vi "Get Channel Groups.vi"(8 "error in":errorcluster, 10 "Channel JSON List":string[](array[string]), 11 "Channel Type List":string[](array[string])) -> (0 "error out":errorcluster, 3 "ChannelGroups":T1)   [LabVIEW 2026, in "Template Deployment Hooks.lvlib"]
uses:
  Template Deployment Hooks.lvlib
  <vilib>/JDP Science/JSONtext/JSONtext.lvlib
  Types/Channel Mode.ctl
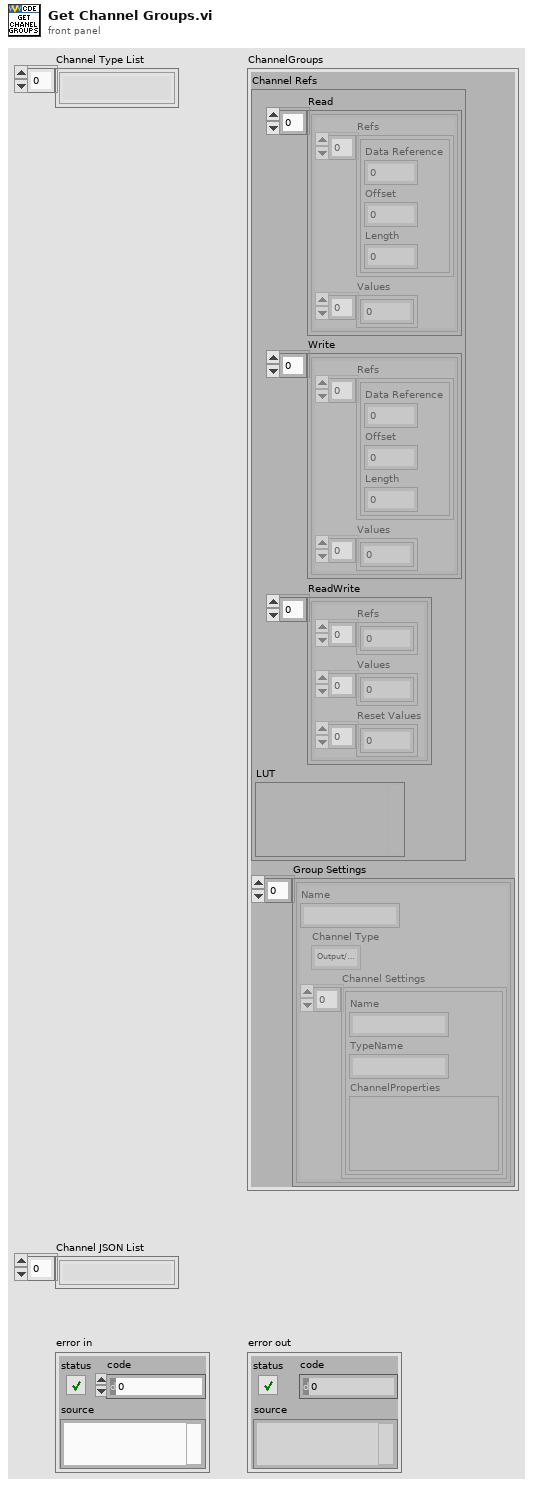
[diagram p1: front panel]
types:
  T1 = cluster{"Channel Refs":cluster{"Read":cluster{"Refs":cluster{"Data Reference":i32, "Offset":u64, "Length":u64}[], "Values":dbl[]}[], "Write":cluster{"Refs":cluster{"Data Reference":i32, "Offset":u64, "Length":u64}[], "Values":dbl[]}[], "ReadWrite":cluster{"Refs":i32[], "Values":dbl[], "Reset Values":dbl[]}[], "LUT":variant}, "Group Settings":cluster{"Name":string, "Channel Type":enum16{"Output/Write", "Input/Read", "Input/ReadWrite"}, "Channel Settings":cluster{"Name":string, "TypeName":string, "ChannelProperties":variant}[]}[]}
  T2 = typedef "Template Deployment Hooks.lvlib/Channel Mode.ctl" = enum16{"Output/Write", "Input/Read", "Input/ReadWrite"}
  T3 = cluster{"Group Name":string, "Channel Type":T2, "Channel DataReferences":i32[]}[]
  T4 = cluster{"Name":string, "Channel Type":enum16{"Output/Write", "Input/Read", "Input/ReadWrite"}, "Channel Settings":cluster{"Name":string, "TypeName":string, "ChannelProperties":variant}[]}[]
  T5 = cluster{"Name":string, "TypeName":string, "ChannelProperties":variant}
  T6 = cluster{"Group Name":string, "Channel Type":T2, "Channel Data References":i32[]}[]
  T7 = cluster{"Read":cluster{"Refs":cluster{"Data Reference":i32, "Offset":u64, "Length":u64}[], "Values":dbl[]}[], "Write":cluster{"Refs":cluster{"Data Reference":i32, "Offset":u64, "Length":u64}[], "Values":dbl[]}[], "ReadWrite":cluster{"Refs":i32[], "Values":dbl[], "Reset Values":dbl[]}[], "LUT":variant}
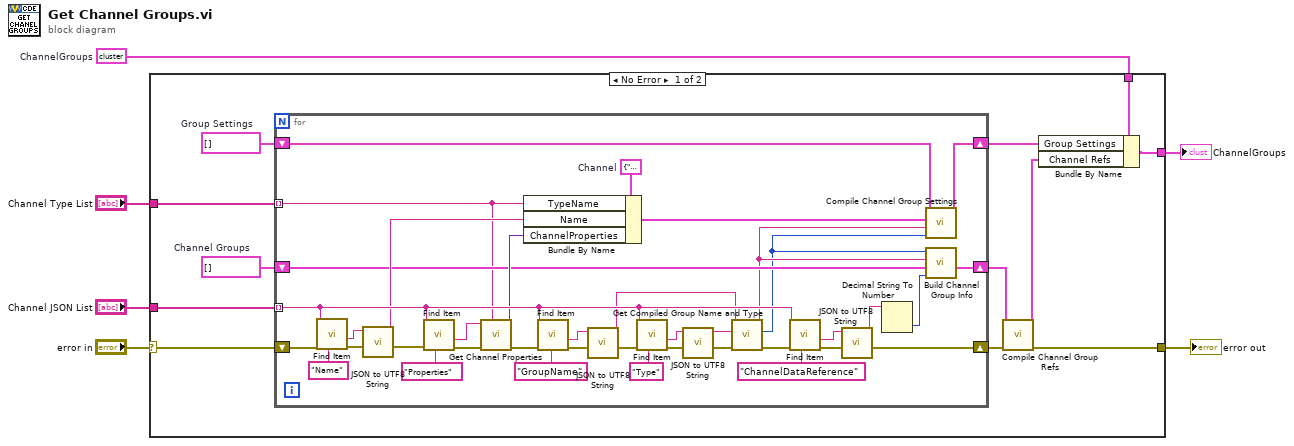
[diagram p0: block diagram]
diagram:
  w1 = T1 {"Channel Refs"={"Read"=[], "Write"=[], "ReadWrite"=[], "LUT"=variant}, "Group Settings"=[]}  # ChannelGroups
  n1 = case shown="No Error" "error in" {
    selector: "error in" -> [w17 w56]
    tunnel: [w18 w56] -> w5
    tunnel: "Channel JSON List" -> [w16 _]
    tunnel: "Channel Type List" -> [w15 _]
    tunnel: [w14 _] -> w2
    tunnel: w1 -> [w7 _]
    frame No Error {
      w8 = T3 []  # Channel Groups
      w12 = T4 []  # Group Settings
      n2 = for {
        shift-right: [w45] -> w13
        shift-left: w17 -> [w55]
        tunnel: w16 -> [w39] mode=indexing
        tunnel: w15 -> [w19] mode=indexing
        shift-right: [w30] -> w10
        shift-left: w12 -> [w31]
        shift-right: [w26] -> w9
        shift-left: w8 -> [w25]
        w35 = T5 {"Name"="", "TypeName"="", "ChannelProperties"=variant}  # Channel
        n3 = call <vilib>:"Find Item.vi"("$Path or Item Name"="Name", "error in (no error)"=w55, "JSON"=w39) -> ("error out"=w54:errorcluster, "<JSON>"=w38:string)  [unwired: 5 in, 2 out]
        n4 = call <vilib>:"JSON to UTF8 String.vi"("error in (no error)"=w54, "JSON"=w38) -> ("error out"=w53:errorcluster, "<UTF8>String"=w32:string)  [unwired: 8 in]
        n5 = call <vilib>:"Find Item.vi"("$Path or Item Name"="Properties", "error in (no error)"=w53, "JSON"=w39) -> ("error out"=w48:errorcluster, "<JSON>"=w29:string)  [unwired: 5 in, 2 out]
        n6 = call "Get Channel Properties.vi"("TypeName"=w19, "error in"=w48, "JSON"=w29) -> ("error out"=w47:errorcluster, "Channel Properties"=w34:variant)  [unwired: 7 in]
        n7 = Bundle By Name(cluster=w35, "TypeName"=w19, "Name"=w32, "ChannelProperties"=w34) -> (w33:T5)
        n8 = call <vilib>:"Find Item.vi"("$Path or Item Name"="GroupName", "error in (no error)"=w47, "JSON"=w39) -> ("error out"=w52:errorcluster, "<JSON>"=w36:string)  [unwired: 5 in, 2 out]
        n9 = call <vilib>:"JSON to UTF8 String.vi"("error in (no error)"=w52, "JSON"=w36) -> ("error out"=w51:errorcluster, "<UTF8>String"=w27:string)  [unwired: 8 in]
        n10 = call <vilib>:"Find Item.vi"("$Path or Item Name"="Type", "error in (no error)"=w51, "JSON"=w39) -> ("error out"=w50:errorcluster, "<JSON>"=w37:string)  [unwired: 5 in, 2 out]
        n11 = call <vilib>:"JSON to UTF8 String.vi"("error in (no error)"=w50, "JSON"=w37) -> ("error out"=w49:errorcluster, "<UTF8>String"=w28:string)  [unwired: 8 in]
        n12 = call "Get Compiled Group Name and Type.vi"("Channel Type"=w28, "Group Name"=w27) -> ("Group Type"=w22:T2, "Computed Group Name"=w24:string)  [unwired: 8 in]
        n13 = call <vilib>:"Find Item.vi"("$Path or Item Name"="ChannelDataReference", "error in (no error)"=w49, "JSON"=w39) -> ("error out"=w46:errorcluster, "<JSON>"=w21:string)  [unwired: 5 in, 2 out]
        n14 = call <vilib>:"JSON to UTF8 String.vi"("error in (no error)"=w46, "JSON"=w21) -> ("error out"=w45:errorcluster, "<UTF8>String"=w20:string)  [unwired: 8 in]
        n15 = Decimal String To Number(string=w20) -> (number=w23:i32)  [unwired: 2 in, 1 out]
        n16 = call "Compile Channel Group Settings.vi"("Channel Type"=w22, "Group Name"=w24, "Channel Settings"=w33, "Group Settings"=w31) -> ("Group Settings"=w30:T4)  [unwired: 7 in]
        n17 = call "Build Channel Group Info.vi"("Channel Data Reference"=w23, "Channel Groups in"=w25, "Group Name"=w24, "Channel Type"=w22) -> ("Channel Groups out"=w26:T6)  [unwired: 7 in]
      }
      n18 = call "Compile Channel Group Refs.vi"("error in"=w13, "Channel Groups in"=w9) -> ("error out"=w18:errorcluster, "Compiled Channel Groupings"=w11:T7)  [unwired: 8 in]
      n19 = Bundle By Name(cluster=w7, "Group Settings"=w10, "Channel Refs"=w11) -> (w14:T1)
    }
    frame Error {
    }
  }
  "error out" <- w5
  "ChannelGroups" <- w2
